vi "FULL ADDER.vi"() -> ()   [LabVIEW 2020]
panel:
  out "?":bool
  out "SUM":bool
  in  "YZ":bool
  in  "Y":bool
  in  "X":bool
  # "CARRY"
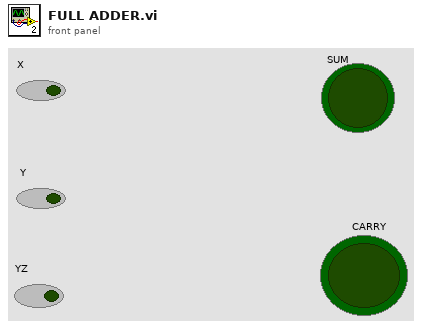
[diagram p1: front panel]
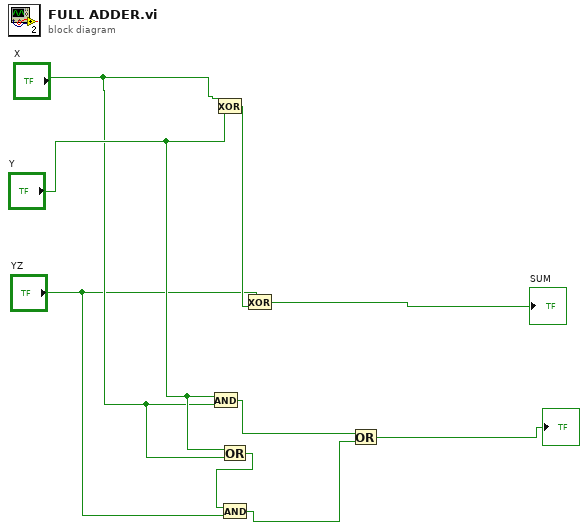
[diagram p0: block diagram]
diagram:
  n1 = And(x="Y", y="X") -> (x .and. y?=w3:bool)
  n2 = Exclusive Or(1:"Y", 2:"X") -> (0:w9:bool)
  n3 = Or(x="Y", y="X") -> (x .or. y?=w5:bool)
  n4 = And(x=w5, y="YZ") -> (x .and. y?=w2:bool)
  n5 = Exclusive Or(1:w9, 2:"YZ") -> (0:→"SUM":bool)
  n6 = Or(x=w3, y=w2) -> (x .or. y?=→"?":bool)
